vi "阶乘的递归算法.vi"(9 "n":u32) -> (1 "n!":u32)   [LabVIEW 2021]
doc: "程序的说明请查看我的bl og： \nhttp://ruanqizhen.spaces.live.com/blog/cns!5852D4F797C53FB6!1832.entry"
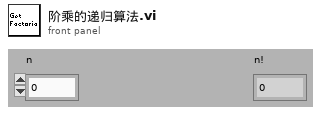
[diagram p1: front panel]
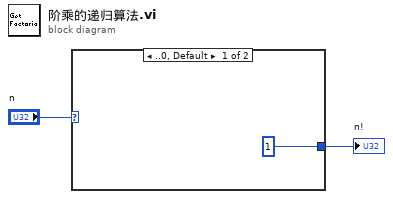
[diagram p0: block diagram]
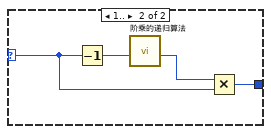
[diagram p2: hidden frame]
diagram:
  n1 = case shown="..0, Default" "n" {
    selector: "n" -> [_ w6]
    tunnel: [u32 1 ("y") w7] -> w2
    frame ..0, Default {
    }
    frame 1.. {
      n2 = Decrement(x=w6) -> (x-1=w5:u32)
      n3 = call "阶乘的递归算法.vi"("n"=w5) -> ("n!"=w4:u32)  [unwired: 10 in]
      n4 = Multiply(x=w4, y=w6) -> (x*y=w7:u32)
    }
  }
  "n!" <- w2
